vi "final.vi"() -> ()   [LabVIEW 2014]
panel:
  in  "?":enum32{"数据处理与显示", "视频图像检测", "性能评价"}(tab)
  in  "串口号":i32
  out "?":i32(graph)
  out "?":u32(graph)
  in  "IP地址":string
  in  "加速度截取":i32
  in  "角度截取":i32
  in  "读取字节数":i32
  in  "Stop":bool
  in  "相机选择":refnum<k21> caption="IMAQdx Session"
  in  "直线类型":u32(ring) items=["Left to Right", "Right to Left", "Top to Bottom", "Bottom to Top"]
  out "?":T1(plugin-control)
  out "?":T1(plugin-control)
  out "直线数目":i32
  out "?":bool
  out "平均速度":dbl
  out "平均速度":dbl
  in  "确定按钮":bool
  in  "?":bool
  out "△加速度":dbl
  out "平均加速度":dbl
  out "评价结果":string
  out "分数总计":dbl
  out "?":dbl
  out "?":dbl
  out "?":dbl
  out "?":dbl
  out "?":dbl
  out "?":dbl
  out "?":dbl
  out "?":dbl
  out "?":dbl
  out "?":dbl
  out "?":dbl
  out "?":dbl
  out "?":dbl
  out "?":dbl
  out "?":dbl
  out "?":dbl
  out "?":dbl
  out "?":dbl
  out "?":dbl
  out "?":dbl
  out "?":dbl
  in  "输入评价结果储存路径":path
  out "?":string
  out "?":bool
  out "?":string
  out "?":bool
  out "?":string
  out "?":bool
  out "?":string
  out "?":bool
  out "?":string
  out "?":bool
  out "?":string
  out "?":bool
  out "?":string
  out "?":bool
  in  "壕沟":dbl=0.15 format="%#_13g"
  in  "断崖":dbl=0.1 format="%#_13g"
  in  "台阶":dbl=0.1 format="%#_13g"
  in  "坡面路":dbl=0.2 format="%#_13g"
  in  "草地路":dbl=0.15 format="%#_13g"
  in  "碎石路":dbl=0.15 format="%#_13g"
  in  "单项考核":dbl=0.15 format="%#_13g"
  out "毫秒计时值":u32
  out "毫秒计时值 2":u32
  out "毫秒计时值 3":u32
  # "机器人运行性能检测与综合评价系统"
  # "视频图像采集"
  # "直线检测"
  # "考核项目权重"
  # "评价指标权重"
  # "系统运行"
  # "考核项目   平均速度   平均加速度  信号指示 项目得分"
  # "单项考核"
  # "单项考核"
  # "路面考核   平均速度     △加速度"
  # "碎石路"
  # "草地路"
  # "坡面路"
  # "路面考核"
  # "障碍考核   起始时间     结束时间"
  # "存储路径"
  # "台阶"
  # "断崖"
  # "壕沟"
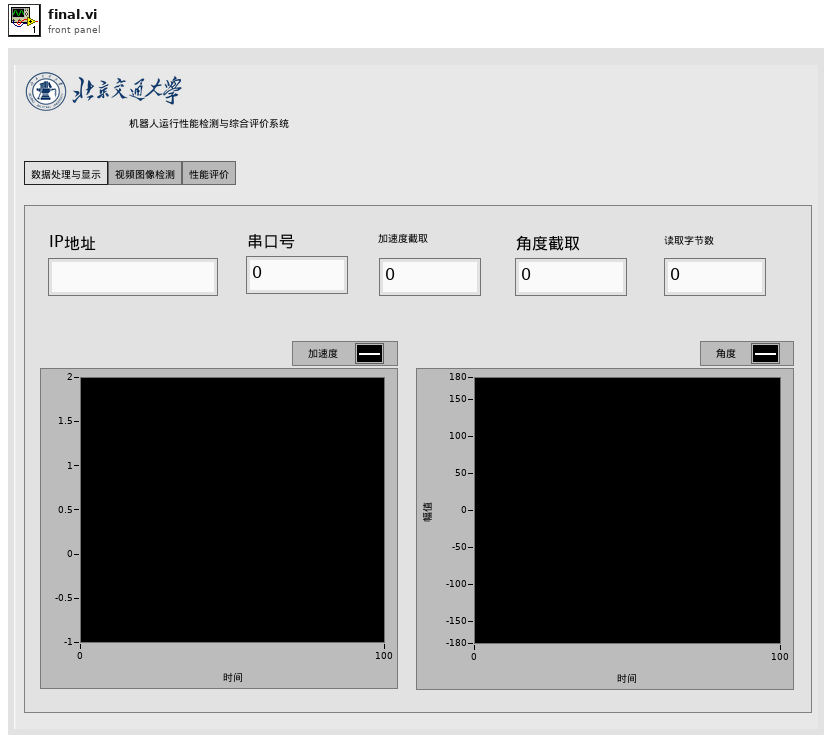
[diagram p1: front panel]
types:
  T1 = typedef "IMAQ Image.ctl" = refnum<image>
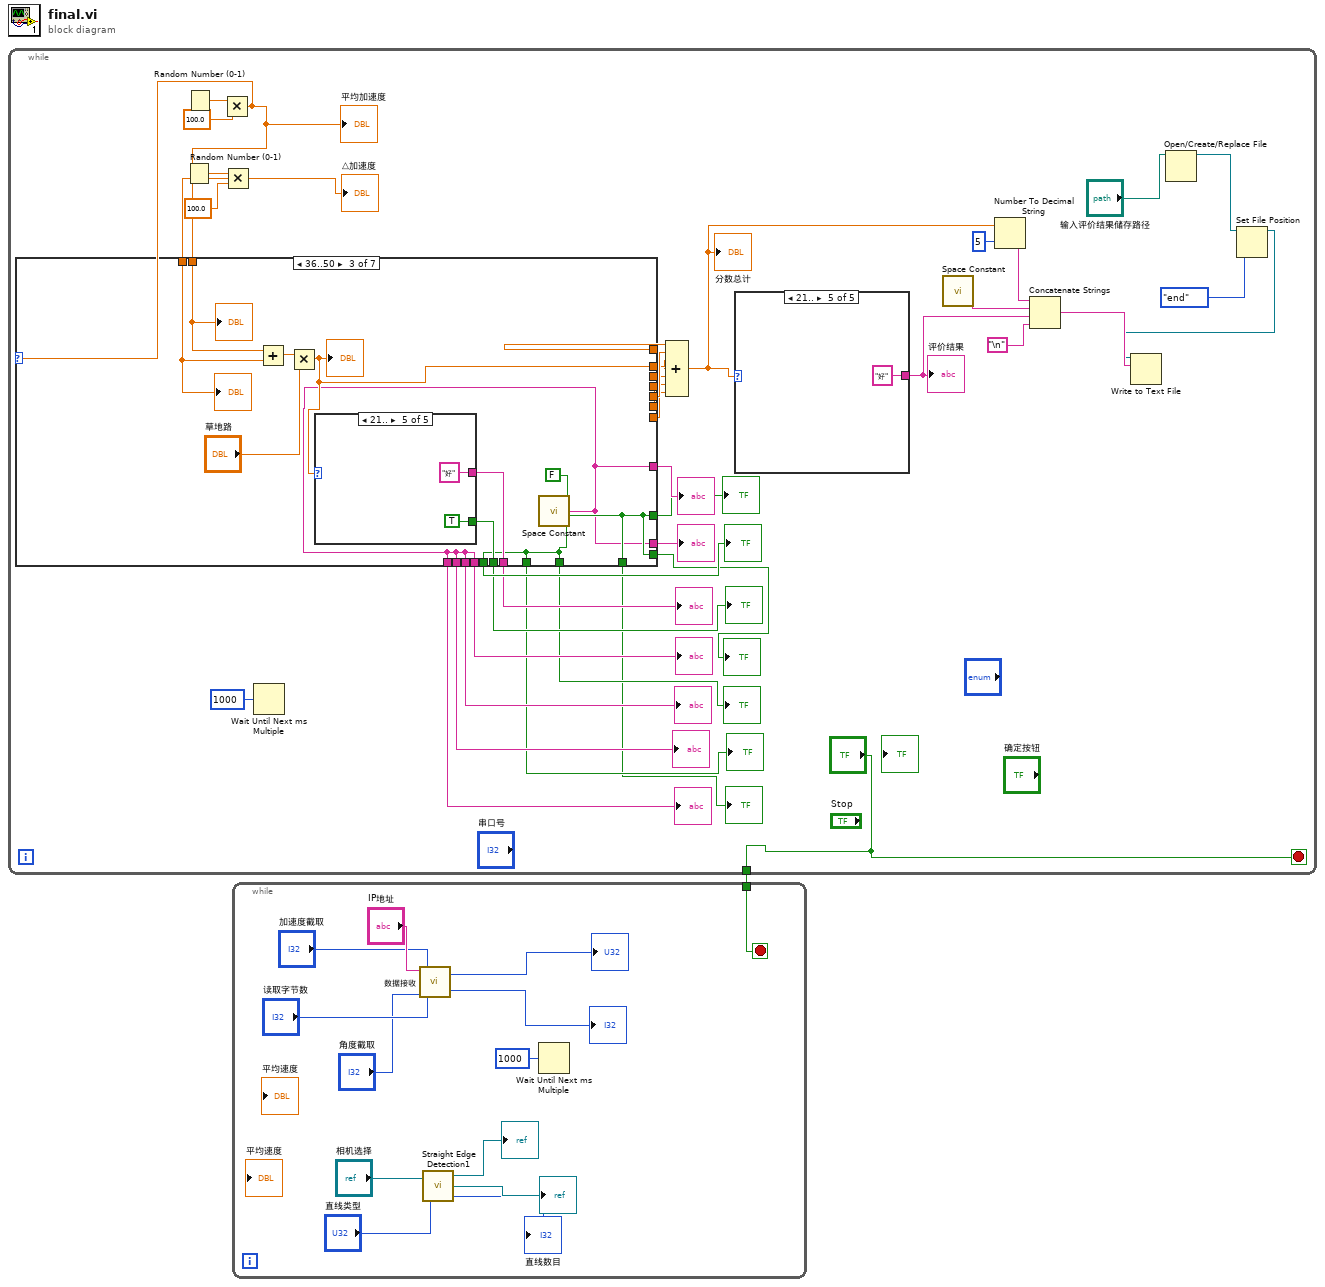
[diagram p0: block diagram]
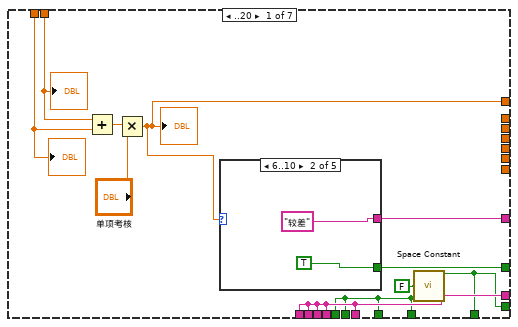
[diagram p2: hidden frame]
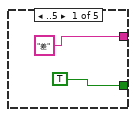
[diagram p3: hidden frame]
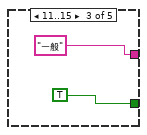
[diagram p4: hidden frame]
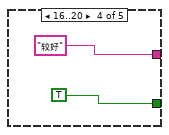
[diagram p5: hidden frame]
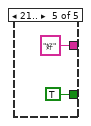
[diagram p6: hidden frame]
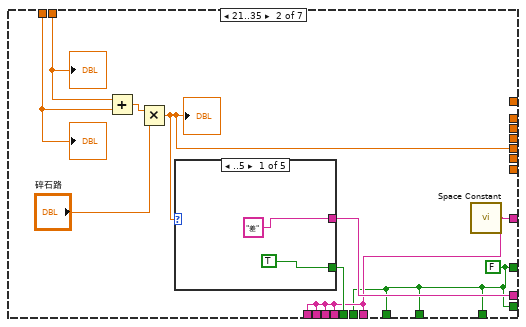
[diagram p7: hidden frame]
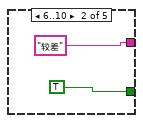
[diagram p8: hidden frame]
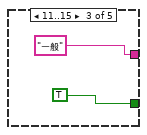
[diagram p9: hidden frame]
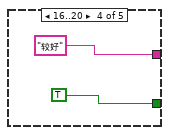
[diagram p10: hidden frame]
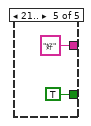
[diagram p11: hidden frame]
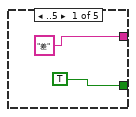
[diagram p12: hidden frame]
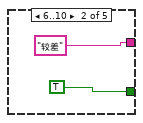
[diagram p13: hidden frame]
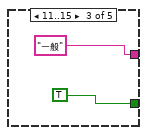
[diagram p14: hidden frame]
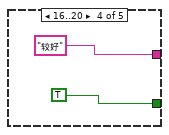
[diagram p15: hidden frame]
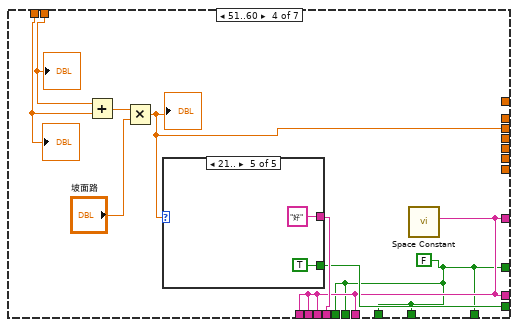
[diagram p16: hidden frame]
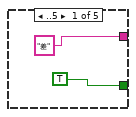
[diagram p17: hidden frame]
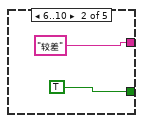
[diagram p18: hidden frame]
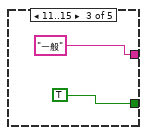
[diagram p19: hidden frame]
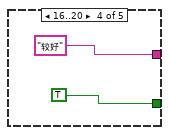
[diagram p20: hidden frame]
diagram:
  n1 = while {
    tunnel: ["?"] -> w1
    stop <- "?" stop-if-true
    n2 = Random Number (0-1)() -> (number: 0 to 1=w31:dbl)
    n3 = Random Number (0-1)() -> (number: 0 to 1=w29:dbl)
    n4 = Multiply(x=w29, y=100.0) -> (x*y=w4:dbl)
    "平均加速度" <- w4
    n5 = Multiply(x=w31, y=100.0) -> (x*y=w3:dbl)
    "△加速度" <- w3
    n6 = case shown="36..50" w4 {
      tunnel: w4 -> [w50 w69 w88 w107 w127 w147 w167]
      tunnel: w3 -> [w49 w68 w87 w106 w126 w146 w166]
      tunnel: [w46 _ _ _ _ _ _] -> w27
      tunnel: [_ w65 _ _ _ _ _] -> w26
      tunnel: [_ _ w84 _ _ _ _] -> w25
      tunnel: [_ _ _ w103 _ _ _] -> w24
      tunnel: [_ _ _ _ w123 _ _] -> w23
      tunnel: [_ _ _ _ _ w143 _] -> w22
      tunnel: [_ _ _ _ _ _ w163] -> w21
      tunnel: [w45 w62 w80 w100 w120 w140 w160] -> w19
      tunnel: [w44 w61 w81 w99 w119 w139 w159] -> w18
      tunnel: [w43 w64 w80 w100 w120 w140 w160] -> w17
      tunnel: [w42 w63 w81 w99 w119 w139 w159] -> w16
      tunnel: [w43 w62 w83 w100 w120 w140 w160] -> w15
      tunnel: [w42 w61 w82 w99 w119 w139 w159] -> w14
      tunnel: [w43 w62 w80 w102 w120 w140 w160] -> w13
      tunnel: [w42 w61 w81 w101 w119 w139 w159] -> w12
      tunnel: [w43 w62 w80 w100 w122 w140 w160] -> w11
      tunnel: [w42 w61 w81 w99 w121 w139 w159] -> w10
      tunnel: [w43 w62 w80 w100 w120 w142 w160] -> w9
      tunnel: [w42 w61 w81 w99 w119 w141 w159] -> w8
      tunnel: [w43 w62 w80 w100 w120 w140 w162] -> w7
      tunnel: [w42 w61 w81 w99 w119 w139 w161] -> w6
      frame ..20 {
        w42 = FALSE
        n7 = Add(x=w50, y=w49) -> (x+y=w48:dbl)
        n8 = Multiply(x=w48, y="单项考核") -> (x*y=w46:dbl)
        "?" <- w46
        n9 = case shown="6..10" w46 {
          tunnel: ["差" "较差" "一般" "较好" "好"] -> w45
          tunnel: [TRUE TRUE TRUE TRUE TRUE] -> w44
          frame ..5 {
          }
          frame 6..10 {
          }
          frame 11..15 {
          }
          frame 16..20 {
          }
          frame 21.. {
          }
        }
        n10 = call <vilib>:"Space Constant.vi"() -> ("String"=w43:string)
        "?" <- w50
        "?" <- w49
      }
      frame 21..35 {
        w61 = FALSE
        n11 = Add(x=w69, y=w68) -> (x+y=w67:dbl)
        n12 = Multiply(x=w67, y="碎石路") -> (x*y=w65:dbl)
        "?" <- w65
        n13 = case shown="..5" w65 {
          tunnel: ["差" "较差" "一般" "较好" "好"] -> w64
          tunnel: [TRUE TRUE TRUE TRUE TRUE] -> w63
          frame ..5 {
          }
          frame 6..10 {
          }
          frame 11..15 {
          }
          frame 16..20 {
          }
          frame 21.. {
          }
        }
        n14 = call <vilib>:"Space Constant.vi"() -> ("String"=w62:string)
        "?" <- w69
        "?" <- w68
      }
      frame 36..50 {
        w81 = FALSE
        n15 = Add(x=w88, y=w87) -> (x+y=w86:dbl)
        n16 = Multiply(x=w86, y="草地路") -> (x*y=w84:dbl)
        "?" <- w84
        n17 = case shown="21.." w84 {
          tunnel: ["差" "较差" "一般" "较好" "好"] -> w83
          tunnel: [TRUE TRUE TRUE TRUE TRUE] -> w82
          frame ..5 {
          }
          frame 6..10 {
          }
          frame 11..15 {
          }
          frame 16..20 {
          }
          frame 21.. {
          }
        }
        n18 = call <vilib>:"Space Constant.vi"() -> ("String"=w80:string)
        "?" <- w88
        "?" <- w87
      }
      frame 51..60 {
        w99 = FALSE
        n19 = Add(x=w107, y=w106) -> (x+y=w105:dbl)
        n20 = Multiply(x=w105, y="坡面路") -> (x*y=w103:dbl)
        "?" <- w103
        n21 = case shown="21.." w103 {
          tunnel: ["差" "较差" "一般" "较好" "好"] -> w102
          tunnel: [TRUE TRUE TRUE TRUE TRUE] -> w101
          frame ..5 {
          }
          frame 6..10 {
          }
          frame 11..15 {
          }
          frame 16..20 {
          }
          frame 21.. {
          }
        }
        n22 = call <vilib>:"Space Constant.vi"() -> ("String"=w100:string)
        "?" <- w107
        "?" <- w106
      }
      frame 61..75 {
        w119 = FALSE
        n23 = Add(x=w127, y=w126) -> (x+y=w125:dbl)
        n24 = Multiply(x=w125, y="台阶") -> (x*y=w123:dbl)
        "?" <- w123
        n25 = case shown="21.." w123 {
          tunnel: ["差" "较差" "一般" "较好" "好"] -> w122
          tunnel: [TRUE TRUE TRUE TRUE TRUE] -> w121
          frame ..5 {
          }
          frame 6..10 {
          }
          frame 11..15 {
          }
          frame 16..20 {
          }
          frame 21.. {
          }
        }
        n26 = Tick Count (ms)() -> (millisecond timer value=→"毫秒计时值":u32)
        n27 = call <vilib>:"Space Constant.vi"() -> ("String"=w120:string)
        "?" <- w127
        "?" <- w126
      }
      frame 76..85 {
        w139 = FALSE
        n28 = Add(x=w147, y=w146) -> (x+y=w145:dbl)
        n29 = Multiply(x=w145, y="断崖") -> (x*y=w143:dbl)
        "?" <- w143
        n30 = case shown="21.." w143 {
          tunnel: ["差" "较差" "一般" "较好" "好"] -> w142
          tunnel: [TRUE TRUE TRUE TRUE TRUE] -> w141
          frame ..5 {
          }
          frame 6..10 {
          }
          frame 11..15 {
          }
          frame 16..20 {
          }
          frame 21.. {
          }
        }
        n31 = Tick Count (ms)() -> (millisecond timer value=→"毫秒计时值 2":u32)
        n32 = call <vilib>:"Space Constant.vi"() -> ("String"=w140:string)
        "?" <- w147
        "?" <- w146
      }
      frame 86.. {
        w159 = FALSE
        n33 = Add(x=w167, y=w166) -> (x+y=w165:dbl)
        n34 = Multiply(x=w165, y="壕沟") -> (x*y=w163:dbl)
        "?" <- w163
        n35 = case shown="21.." w163 {
          tunnel: ["差" "较差" "一般" "较好" "好"] -> w162
          tunnel: [TRUE TRUE TRUE TRUE TRUE] -> w161
          frame ..5 {
          }
          frame 6..10 {
          }
          frame 11..15 {
          }
          frame 16..20 {
          }
          frame 21.. {
          }
        }
        n36 = Tick Count (ms)() -> (millisecond timer value=→"毫秒计时值 3":u32)
        n37 = call <vilib>:"Space Constant.vi"() -> ("String"=w160:string)
        "?" <- w167
        "?" <- w166
      }
    }
    "?" <- w18
    "?" <- w19
    "?" <- w17
    "?" <- w16
    "?" <- w15
    "?" <- w14
    "?" <- w13
    "?" <- w12
    "?" <- w11
    "?" <- w10
    "?" <- w9
    "?" <- w8
    "?" <- w7
    "?" <- w6
    n38 = Wait Until Next ms Multiple(millisecond multiple=u32 1000 ("毫秒倍数")) -> ()  [unwired: 1 out]
    n39 = Compound Arithmetic op=ADD(w27, w26, w25, w24, w23, w22, w21) -> (w20:dbl)
    "分数总计" <- w20
    n40 = case shown="21.." w20 {
      tunnel: ["差" ("字符串") "较差" ("字符串") "一般" ("字符串") "较好" ("字符串") "好" ("字符串")] -> w38
      frame 0..5, Default {
      }
      frame 6..10 {
      }
      frame 11..15 {
      }
      frame 16..20 {
      }
      frame 21.. {
      }
    }
    "评价结果" <- w38
    n41 = call <vilib>:"Space Constant.vi"() -> ("String"=w39:string)
    n42 = Number To Decimal String(number=w20, width (-)=i16 5 ("宽度(-)")) -> (decimal integer string=w40:string)
    n43 = Concatenate Strings(w40, w39, w38, "\n") -> (w37:string)
    n44 = Open/Create/Replace File(file path (use dialog)="输入评价结果储存路径") -> (refnum out=w32:refnum<file>)  [unwired: 5 in, 2 out]
    n45 = Set File Position(refnum=w32, from (0:start)=enum16{"start", "end", "current"}."end" ("自（0:起始）")) -> (refnum out=w34:refnum<file>)  [unwired: 2 in, 1 out]
    n46 = Write to Text File(file (use dialog)=w34, text=w37) -> ()  [unwired: 2 in, 3 out]
  }
  n47 = while {
    tunnel: w1 -> [w183]
    stop <- w183 stop-if-true
    n48 = call "数据接收.vi"("角加速度截取长度"="角度截取", "读取字节数"="读取字节数", "加速度截取长度"="加速度截取", "IP地址"="IP地址") -> ("角加速度"=→"?":i32, "加速度"=→"?":u32)
    n49 = call "Straight Edge Detection1.vi"("Camera Name"="相机选择", "Search Direction"="直线类型") -> ("采集视频"=→"?":T1, "边缘检测（右键单击图像Zoom to Fit还原图像）"=→"?":T1, "Numbers of lines(Red)"=→"直线数目":i32)
    n50 = Wait Until Next ms Multiple(millisecond multiple=u32 1000 ("毫秒倍数")) -> ()  [unwired: 1 out]
  }
